vi "Start Server.vi"(5 "Server Key File (.key)":path, 7 "Server Certificate File (.crt)":path, 8 "error in (no error)":errorcluster, 10 "gRPCid":T1, 11 "Server Address":string) -> (0 "error out":errorcluster)   [LabVIEW 2020, in "server12.lvlib" / "gprc-lvsupport.lvlib"]
uses:
  gprc-lvsupport.lvlib
  typeDefs/grpcId.ctl
  <vilib>/Utility/error.llb/Error Cluster From Error Code.vi
  <vilib>/ErrorRing/Error Ring.xnode
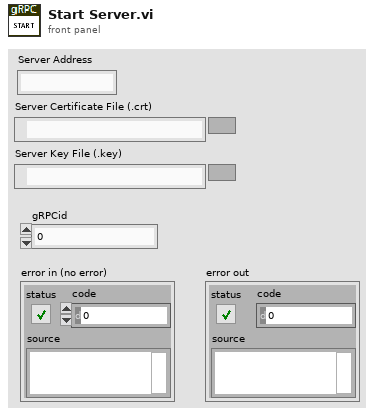
[diagram p1: front panel]
types:
  T1 = typedef "server12.lvlib/gprc-lvsupport.lvlib/grpcId.ctl" = u64
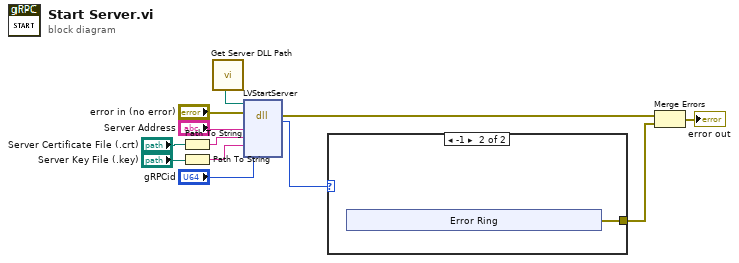
[diagram p0: block diagram]
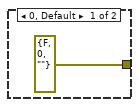
[diagram p2: hidden frame]
diagram:
  n1 = Path To String(path="Server Certificate File (.crt)") -> (string=w9:string)
  n2 = Path To String(path="Server Key File (.key)") -> (string=w8:string)
  n3 = call "Get Server DLL Path.vi"() -> ("Server dll path"=w1:path)
  n4 = dll-call lib="C:/Users/XEnderMD/Desktop/LV gRPC/labview source/gRPC interface/dlls/labview_grpc_server.dll" fn="LVStartServer"(path in=w1, error in="error in (no error)", "serveraddress"="Server Address", "serverCertificateFile"=w9, "serverKeyFile"=w8, "serverid"="gRPCid") -> (error out=w2:errorcluster, "return type"=w5:i32)  [unwired: 5 in, 1 out]
  n5 = case shown="-1" w5 {
    tunnel: [errorcluster {"status"=FALSE, "code"=0, "source"=""} ("error constant") w14] -> w3
    frame 0, Default {
    }
    frame -1 {
      n6 = xnode "Error Ring"() -> ("error out"=w14:errorcluster)
    }
  }
  n7 = Merge Errors(w2, w3) -> (→"error out":errorcluster)
